vi "Protected Data Channel.vi"(8 "error in (no error)":errorcluster, 11 "Node Ptr":T1 format="%.0x") -> (0 "error out":errorcluster)   [LabVIEW 2019, in "Ghost Bus Addon System Explorer.lvlib"]
uses:
  <vilib>/NI VeriStand/Custom Device API/Custom Device Item Ref.ctl
  Ghost Bus Addon System Explorer.lvlib
  <vilib>/NI VeriStand/Custom Device API/Custom Device API.lvlib
panel:
  in  "Default Value":dbl
  in  "Header":cluster{"Section Name":string}={"Section Name"="Signal Settings"}
  in  "Description":string
  out "Name":string
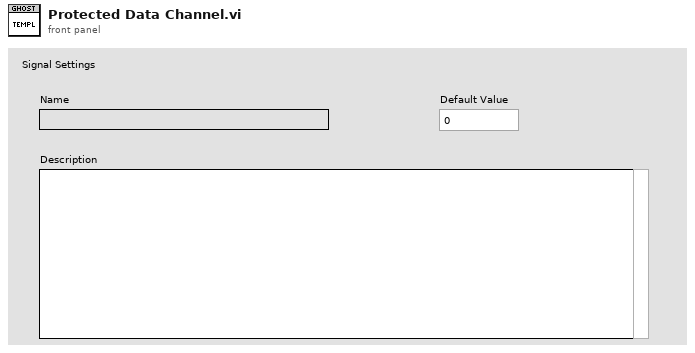
[diagram p1: front panel]
types:
  T1 = typedef "Custom Device API.lvlib/Custom Device Item Ref.ctl" = u64
  T2 = typedef "Custom Device API.lvlib/Custom Device Channel.ctl" = cluster{"Type":T3, "Units":string, "Default Value":dbl, "Faultable":bool, "Scalable":bool}
  T3 = typedef "Custom Device API.lvlib/Custom Device Channel Type.ctl" = enum16{"Input", "Output"}
  T4 = typedef "Custom Device API.lvlib/Custom Device Item Info.ctl" = cluster{"Name":string, "Is Channel":bool, "GUID":string, "Is Waveform":bool}
  T5 = typedef "Custom Device API.lvlib/Custom Device Commands.ctl" = enum16{"Default", "Item renamed", "Shutdown", "Dynamic button pressed"}
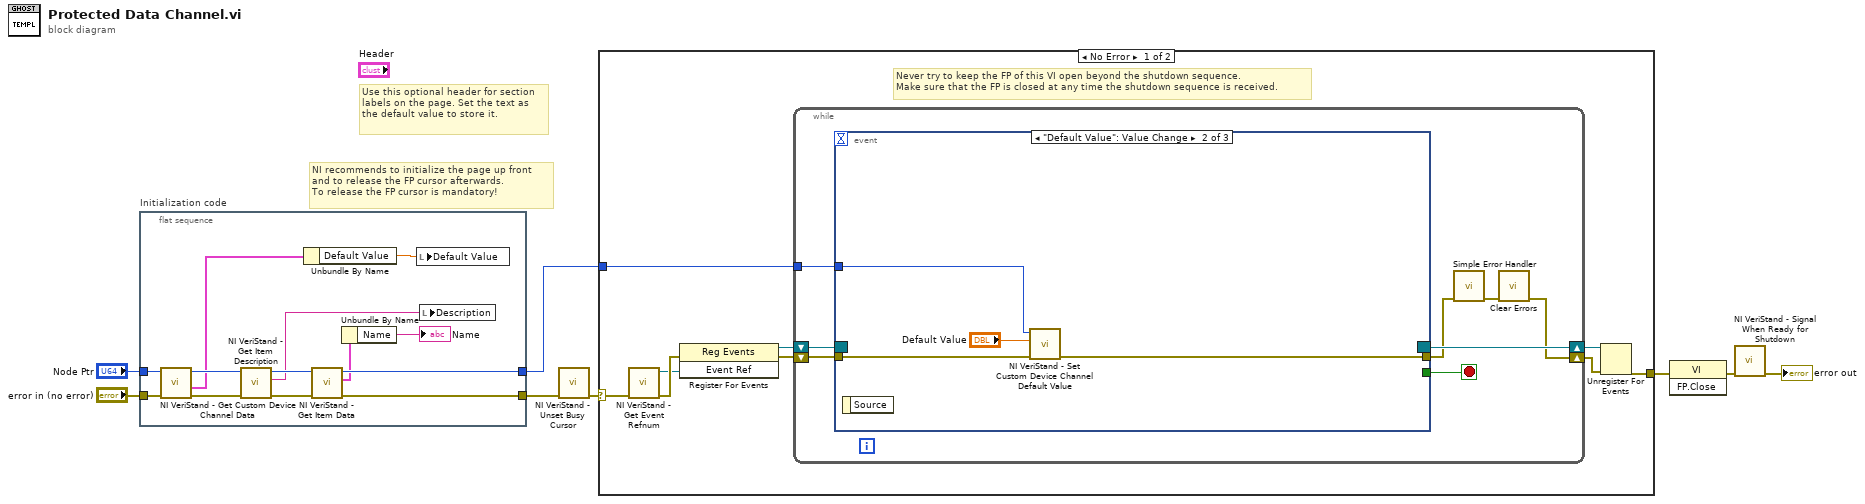
[diagram p0: block diagram]
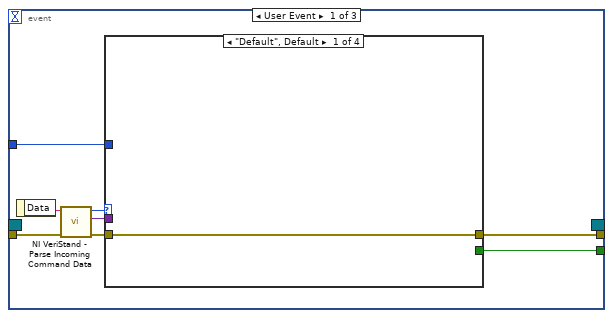
[diagram p2: hidden frame]
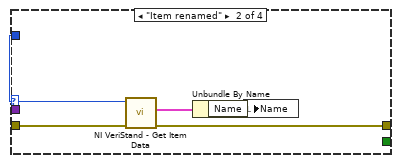
[diagram p3: hidden frame]
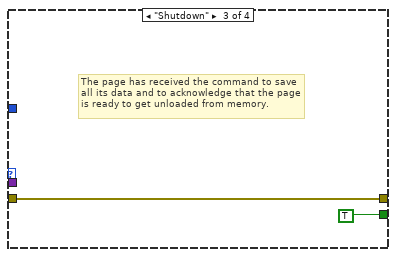
[diagram p4: hidden frame]
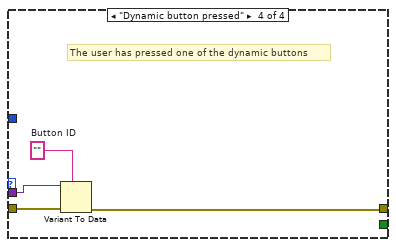
[diagram p5: hidden frame]
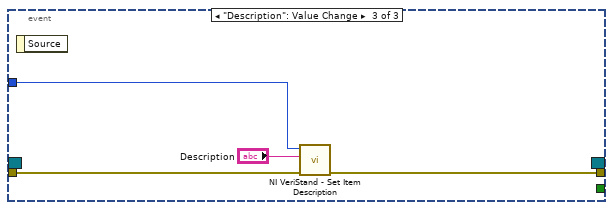
[diagram p6: hidden frame]
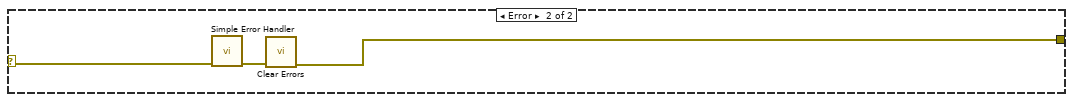
[diagram p7: hidden frame]
diagram:
  # "Use this optional header for section labels on the page. Set the text as the default value to store it."
  # "NI recommends to initialize the page up front\nand to release the FP cursor afterwards.\nTo release the FP cursor is mandatory!"
  n1 = flat-sequence "Initialization code" {
    tunnel: "error in (no error)" -> [w13]
    tunnel: "Node Ptr" -> [w15]
    tunnel: [w16] -> w4
    tunnel: [w21] -> w1
    frame #0 {
      n2 = call <vilib>:"NI VeriStand - Get Custom Device Channel Data.vi"("error in (no error)"=w13, "Channel Ref in"=w15) -> ("error out"=w12:errorcluster, "Channel"=w11:T2, "Channel Ref out"=w14:T1)  [unwired: 4 in, 3 out]
      n3 = call <vilib>:"NI VeriStand - Get Item Description.vi"("error in (no error)"=w12, "Item Ref in"=w14) -> ("error out"=w18:errorcluster, "Description"=w19:string, "Item Ref out"=w20:T1)  [unwired: 7 out]
      n4 = Unbundle By Name(w11) -> ("Default Value"=w10:dbl)
      n5 = call <vilib>:"NI VeriStand - Get Item Data.vi"("error in (no error)"=w18, "Item Ref in"=w20) -> ("error out"=w16:errorcluster, "Item Info"=w17:T4, "Item Ref out"=w21:T1)  [unwired: 7 out]
      n6 = Unbundle By Name(w17) -> ("Name"=→"Name":string)
      n7 = local write "Default Value"(w10) -> ()
      n8 = local write "Description"(w19) -> ()
    }
  }
  n9 = call <vilib>:"NI VeriStand - Unset Busy Cursor.vi"("error in (no error)"=w4) -> ("error out"=w3:errorcluster)  [unwired: 10 out]
  n10 = case shown="No Error" w3 {
    selector: w3 -> [w22 w69]
    tunnel: [w27 w67] -> w8
    tunnel: w1 -> [w23 _]
    frame No Error {
      # "Never try to keep the FP of this VI open beyond the shutdown sequence.\nMake sure that the FP is closed at any time the shutdown sequence is received."
      n11 = call <vilib>:"NI VeriStand - Get Event Refnum.vi"("error in (no error)"=w22) -> ("error out"=w30:errorcluster, "Event Ref"=w26:refnum<user-event>)  [unwired: 9 out]
      n12 = register-events(error in=w30, w26) -> (reference out=w24:refnum<event-registration>, error out=w25:errorcluster)  [unwired: 1 in]
      n13 = while {
        tunnel: w23 -> [w34]
        shift-right: [w31] -> w28
        shift-left: w25 -> [w37]
        shift-right: [w38] -> w29
        shift-left: w24 -> [w36]
        stop <- w35 stop-if-true
        n14 = event shown="[1] \"Default Value\": Value Change" {
          selector: w36 -> [_ _ _]
          dyn-events: [_ _ _] -> w38
          timeout: _ -> [_ _ _]
          tunnel: w37 -> [w46 w62 w65]
          tunnel: [w42 _ _] -> w35
          tunnel: [w41 w60 w64] -> w33
          tunnel: w34 -> [w40 w61 w66]
          event User Event {
            n15 = event-data() -> ("Data"=w45:string)  [unwired: 1 out]
            n16 = call <vilib>:"NI VeriStand - Parse Incoming Command Data.vi"("error in (no error)"=w46, "Incoming data"=w45) -> ("error out"=w44:errorcluster, "Outgoing data"=w39:variant, "Action"=w43:T5)  [unwired: 7 out]
            n17 = case shown="\"Default\", Default" w43 {
              tunnel: w44 -> [w47 w52 w53 w58]
              tunnel: [_ _ TRUE _] -> w42
              tunnel: [w47 w49 w53 w55] -> w41
              tunnel: w40 -> [_ w51 _ _]
              tunnel: w39 -> [_ _ _ w57]
              frame "Default", Default {
              }
              frame "Item renamed" {
                n18 = call <vilib>:"NI VeriStand - Get Item Data.vi"("error in (no error)"=w52, "Item Ref in"=w51) -> ("error out"=w49:errorcluster, "Item Info"=w50:T4)  [unwired: 8 out]
                n19 = Unbundle By Name(w50) -> ("Name"=w48:string)
                n20 = local write "Name"(w48) -> ()
              }
              frame "Shutdown" {
                # "The page has received the command to save all its data and to acknowledge that the page is ready to get unloaded from memory."
              }
              frame "Dynamic button pressed" {
                w56 = ""  # Button ID
                # "The user has pressed one of the dynamic buttons"
                n21 = Variant To Data(error in=w58, type=w56, Variant=w57) -> (error out=w55:errorcluster)  [unwired: 1 out]
              }
            }
          }
          event "Default Value": Value Change {
            n22 = event-data() -> ()  [unwired: 2 out]
            n23 = call <vilib>:"NI VeriStand - Set Custom Device Channel Default Value.vi"("error in (no error)"=w62, "Default Value"="Default Value", "Channel Ref in"=w61) -> ("error out"=w60:errorcluster)  [unwired: 7 in, 1 out]
          }
          event "Description": Value Change {
            n24 = event-data() -> ()  [unwired: 2 out]
            n25 = call <vilib>:"NI VeriStand - Set Item Description.vi"("error in (no error)"=w65, "Description"="Description", "Item Ref in"=w66) -> ("error out"=w64:errorcluster)  [unwired: 8 out]
          }
        }
        n26 = call <vilib>:"Simple Error Handler.vi"("error in (no error)"=w33) -> ("error out"=w32:errorcluster)  [unwired: 1 in, 7 out]
        n27 = call <vilib>:"Clear Errors.vi"("error in (no error)"=w32) -> ("error out"=w31:errorcluster)  [unwired: 1 in, 5 out]
      }
      n28 = Unregister For Events(event registration refnum=w29, error in=w28) -> (error out=w27:errorcluster)
    }
    frame Error {
      n29 = call <vilib>:"Simple Error Handler.vi"("error in (no error)"=w69) -> ("error out"=w68:errorcluster)  [unwired: 1 in, 7 out]
      n30 = call <vilib>:"Clear Errors.vi"("error in (no error)"=w68) -> ("error out"=w67:errorcluster)  [unwired: 1 in, 5 out]
    }
  }
  n31 = invoke class="VI" method="FP.Close"(error in=w8) -> (error out=w7:errorcluster)  [unwired: 2 in, 2 out]
  n32 = call <vilib>:"NI VeriStand - Signal When Ready for Shutdown.vi"("error in (no error)"=w7) -> ("error out"=→"error out":errorcluster)  [unwired: 10 out]
